vi "Emu_CoreDAQ_Globle.vi"() -> ()   [LabVIEW 2012]
panel:
  in  "Period":dbl=10.0
  out "Enable":bool=TRUE
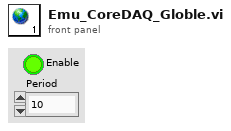
[diagram p1: front panel]
diagram:
